vi "Object Tracking_Example.vi"() -> ()   [LabVIEW 2017]
doc: "This example demonstrates the Traditional MeanShift algorithm to track an object in the image."
uses:
  <vilib>/NI_Real-Time Target Support.lvlib
panel:
  out "CPU Load":dbl(graph)
  in  "AVI File Path":path=path "/home/lvuser/Traffic.avi"
  in  "Stop":bool
  in  "Delay (s.)":dbl(slide)=0.2040816326530612 scale=0.0..2.0
  out "Image":T1(plugin-control)
  # "Overview: Demonstrate the Traditional MeanShift algorithm to track an object in the image.\nRequirements: LabVIEW Full Development System and Vision Development Module.\nInstructions: Run the VI."
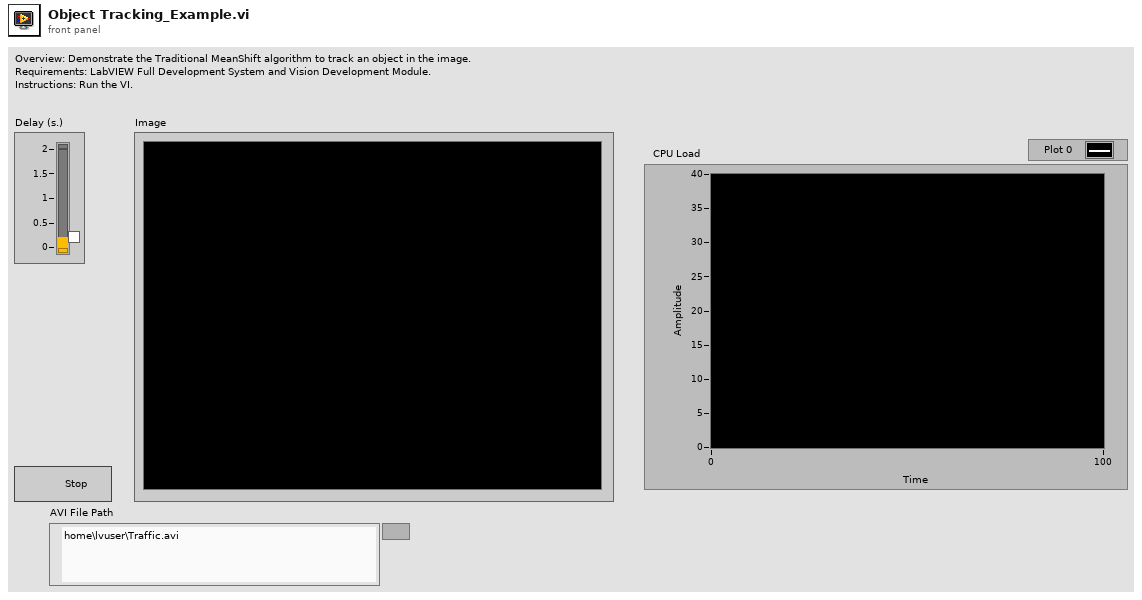
[diagram p1: front panel]
types:
  T1 = typedef "IMAQ Image.ctl" = refnum<image>
  T2 = cluster{"Number of Histogram Bins":i32, "Blending Parameter (%)":dbl, "Maximum Iterations":i32}
  T3 = typedef "Image Type" = u32
  T4 = typedef "IMAQ Object Tracking Session.ctl" = refnum<k20>
  T5 = typedef "IMAQ AVI2 Refnum.ctl" = refnum<k20>
  T6 = typedef "IMAQ Rectangle" = cluster{"Left":i32, "Top":i32, "Right":i32, "Bottom":i32, "Rotation":dbl}
  T7 = typedef "ROI Descriptor" = cluster{"Global Rectangle":i32[], "Contours":cluster{"ID":enum32{"External", "Internal"}, "Type":u32, "Coordinates":i32[]}[]}
  T8 = cluster{"Label":string, "Score":i32, "Angle":dbl, "Location":cluster{"X":dbl, "Y":dbl}, "Bounding Box":cluster{"X":dbl, "Y":dbl}[], "Object Found?":bool}[]
  T9 = cluster{"Label":string, "Score":i32, "Angle":dbl, "Location":cluster{"X":dbl, "Y":dbl}, "Bounding Box":cluster{"X":dbl, "Y":dbl}[], "Object Found?":bool}
  T10 = typedef "NI_Real-Time Target Support.lvlib/RT CPU Load.ctl" = cluster{"Total (%)":dbl, "Time Critical (%)":dbl, "Timed Structures (%)":dbl, "High (%)":dbl, "Above Normal (%)":dbl, "Normal (%)":dbl, "Background (%)":dbl, "Idle (%)":dbl, "ISR (%)":dbl}
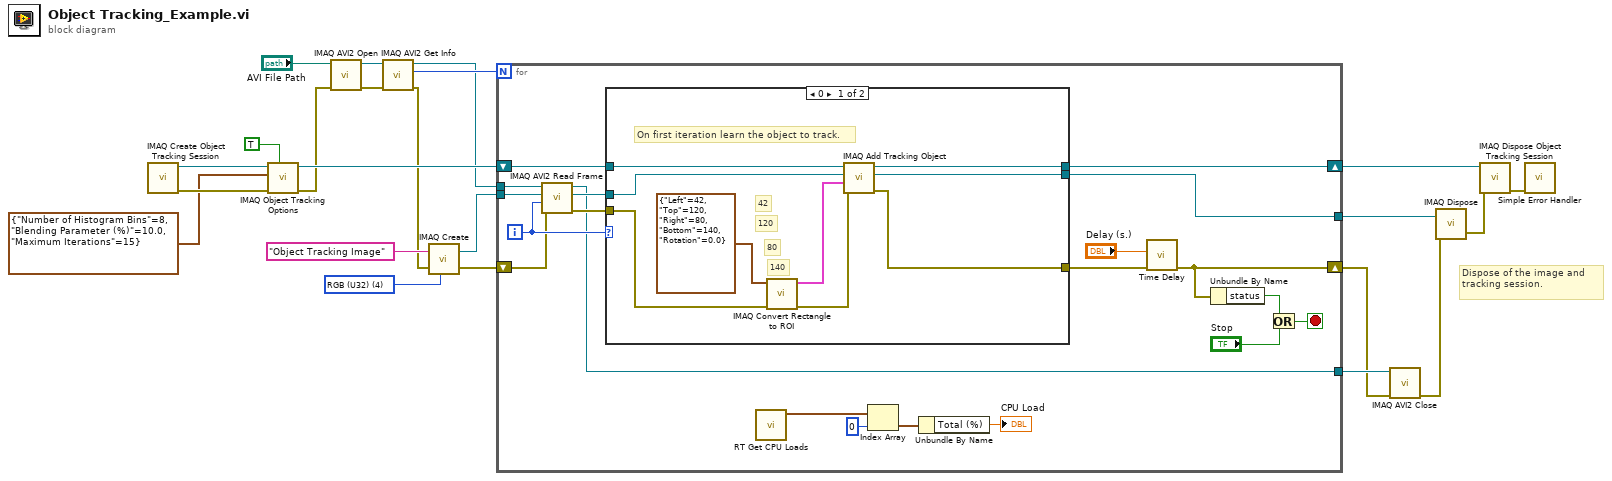
[diagram p0: block diagram]
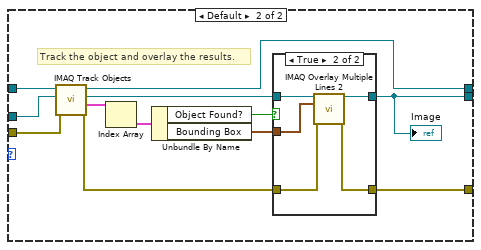
[diagram p2: hidden frame]
diagram:
  w9 = T3 4 items=["Grayscale (U8)", "Grayscale (I16)", "Grayscale (SGL)", "Complex (CSG)", "RGB (U32)", "HSL (U32)", "RGB (U64)", "Grayscale (U16)"] ("Image Type")
  # "Dispose of the image and tracking session."
  n1 = call "IMAQ Create Object Tracking Session"() -> ("error out"=w16:errorcluster, "Object Tracking Session"=w19:T4)  [unwired: 1 in, 9 out]
  n2 = call-poly "IMAQ Object Tracking Options"("Get/Set (Get)"=TRUE, "error in (no error)"=w16, "Mean Shift Options in"=T2 {"Number of Histogram Bins"=8, "Blending Parameter (%)"=10.0, "Maximum Iterations"=15}, "Object Tracking Session In"=w19) -> ("error out"=w15:errorcluster, "Object Tracking Session Out"=w18:T4)  [unwired: 5 in, 1 out]
  n3 = call "IMAQ AVI2 Open"("error in (no error)"=w15, "AVI File Path"="AVI File Path") -> ("error out"=w13:errorcluster, "AVI Refnum"=w14:T5)  [unwired: 8 in]
  n4 = call "IMAQ AVI2 Get Info"("error in (no error)"=w13, "AVI Refnum"=w14) -> ("error out"=w10:errorcluster, "Number of Frames"=w12:u32, "AVI Refnum (duplicate)"=w8:T5)  [unwired: 5 in, 2 out]
  n5 = call "IMAQ Create"("Image Name"="Object Tracking Image", "Image Type"=w9, "error in (no error)"=w10) -> ("New Image"=w7:T1, "error out"=w6:errorcluster)  [unwired: 2 in]
  n6 = for {
    N: w12 -> [_]
    tunnel: [w42] -> w23
    shift-right: [w40] -> w22
    shift-left: w18 -> [w41]
    tunnel: w8 -> [w37]
    tunnel: w7 -> [w36]
    shift-right: [w29] -> w4
    shift-left: w6 -> [w30]
    tunnel: [w28] -> w5
    i -> [w33]
    stop <- w31 stop-if-true
    n7 = call "IMAQ AVI2 Read Frame"("error in (no error)"=w30, "Frame Number"=w33, "Image"=w36, "AVI Refnum"=w37) -> ("error out"=w34:errorcluster, "Image Out"=w35:T1, "AVI Refnum (duplicate)"=w28:T5)  [unwired: 5 in]
    n8 = case shown="0" w33 {
      tunnel: [w49 w64] -> w40
      tunnel: [w51 w61] -> w42
      tunnel: [w50 w57] -> w38
      tunnel: w41 -> [w52 w59]
      tunnel: w35 -> [w48 w55]
      tunnel: w34 -> [w47 w54]
      frame 0 {
        # "140"
        # "80"
        # "42"
        # "120"
        # "On first iteration learn the object to track."
        n9 = call "IMAQ Convert Rectangle to ROI"("error in (no error)"=w47, "Rectangle"=T6 {"Left"=42, "Top"=120, "Right"=80, "Bottom"=140, "Rotation"=0.0}) -> ("error out"=w46:errorcluster, "ROI Descriptor"=w45:T7)  [unwired: 7 in]
        n10 = call "IMAQ Add Tracking Object"("error in (no error)"=w46, "ROI Descriptor"=w45, "Image"=w48, "Object Tracking Session In"=w52) -> ("error out"=w50:errorcluster, "Image (duplicate)"=w51:T1, "Object Tracking Session Out"=w49:T4)  [unwired: 1 in, 4 out]
      }
      frame Default {
        # "Track the object and overlay the results."
        n11 = call "IMAQ Track Objects"("error in (no error)"=w54, "Image"=w55, "Object Tracking Session In"=w59) -> ("error out"=w58:errorcluster, "Objects (pixel)"=w63:T8, "Image (duplicate)"=w62:T1, "Object Tracking Session Out"=w64:T4)  [unwired: 1 in, 4 out]
        n12 = Index Array(array=w63) -> (element=w56:T9)  [unwired: 1 in]
        n13 = Unbundle By Name(w56) -> ("Object Found?"=w53:bool, "Bounding Box"=w60:cluster{"X":dbl, "Y":dbl}[])
        n14 = case shown="True" w53 {
          tunnel: w62 -> [w65 w71]
          tunnel: [w65 w70] -> w61
          tunnel: w60 -> [_ w69]
          tunnel: w58 -> [w66 w68]
          tunnel: [w66 w67] -> w57
          frame False {
          }
          frame True {
            n15 = call "IMAQ Overlay Multiple Lines 2"("Image"=w71, "Line End Points"=w69, "error in (no error)"=w68) -> ("Image Out"=w70:T1, "error out"=w67:errorcluster)  [unwired: 5 in, 6 out]
          }
        }
        "Image" <- w61
      }
    }
    n16 = call <vilib>:"RT Get CPU Loads.vi"() -> ("CPU loads"=w25:T10[])  [unwired: 10 in, 1 out]
    n17 = Index Array(array=w25, index=0) -> (element=w26:T10)
    n18 = Unbundle By Name(w26) -> ("Total (%)"=→"CPU Load":dbl)
    n19 = call "Time Delay"("error in (no error)"=w38, "Delay Time (s)"="Delay (s.)") -> ("error out"=w29:errorcluster)  [unwired: 9 in]
    n20 = Unbundle By Name(w29) -> ("status"=w43:bool)
    n21 = Or(x=w43, y="Stop") -> (x .or. y?=w31:bool)
  }
  n22 = call "IMAQ AVI2 Close"("error in (no error)"=w4, "AVI Refnum"=w5) -> ("error out"=w3:errorcluster)  [unwired: 9 in]
  n23 = call "IMAQ Dispose"("Image"=w23, "error in (no error)"=w3) -> ("error out"=w21:errorcluster)  [unwired: 1 in, 3 out]
  n24 = call "IMAQ Dispose Object Tracking Session"("error in (no error)"=w21, "Object Tracking Session"=w22) -> ("error out"=w20:errorcluster)  [unwired: 9 out]
  n25 = call <vilib>:"Simple Error Handler.vi"("error in (no error)"=w20) -> ()  [unwired: 1 in, 8 out]
